vi "MS_Var_to_Comm_Binary.vi"(11 "Boolean":bool) -> (1 "Array":T3[](array[typedef]) {"CROB value"."Control" items=["Nul"=0, "Pulse On"=1, "Pulse Off"=2, "Latch On"=3, "Latch Off"=4, "Close"=65, "Trip"=129]})   [LabVIEW 2016, in "DNP3_Master_Station_Template.lvlib"]
uses:
  DNP3_Master_Station_Template.lvlib
  <vilib>/DNP3/DNP3_Master/Crob With Index.ctl
  <vilib>/DNP3/DNP3_Common/crob.ctl
  <vilib>/DNP3/DNP3_Common/crob_ctrl.ctl
  <vilib>/Utility/file.llb/Read Delimited Spreadsheet (string).vi
  <vilib>/DNP3/DNP3_Common.lvlib
  <vilib>/DNP3/DNP3_Master.lvlib
panel:
  in  "CROB value":T1 {"Control" items=["Nul"=0, "Pulse On"=1, "Pulse Off"=2, "Latch On"=3, "Latch Off"=4, "Close"=65, "Trip"=129]}
  in  "CROB with point index":T3 {"CROB value"."Control" items=["Nul"=0, "Pulse On"=1, "Pulse Off"=2, "Latch On"=3, "Latch Off"=4, "Close"=65, "Trip"=129]}
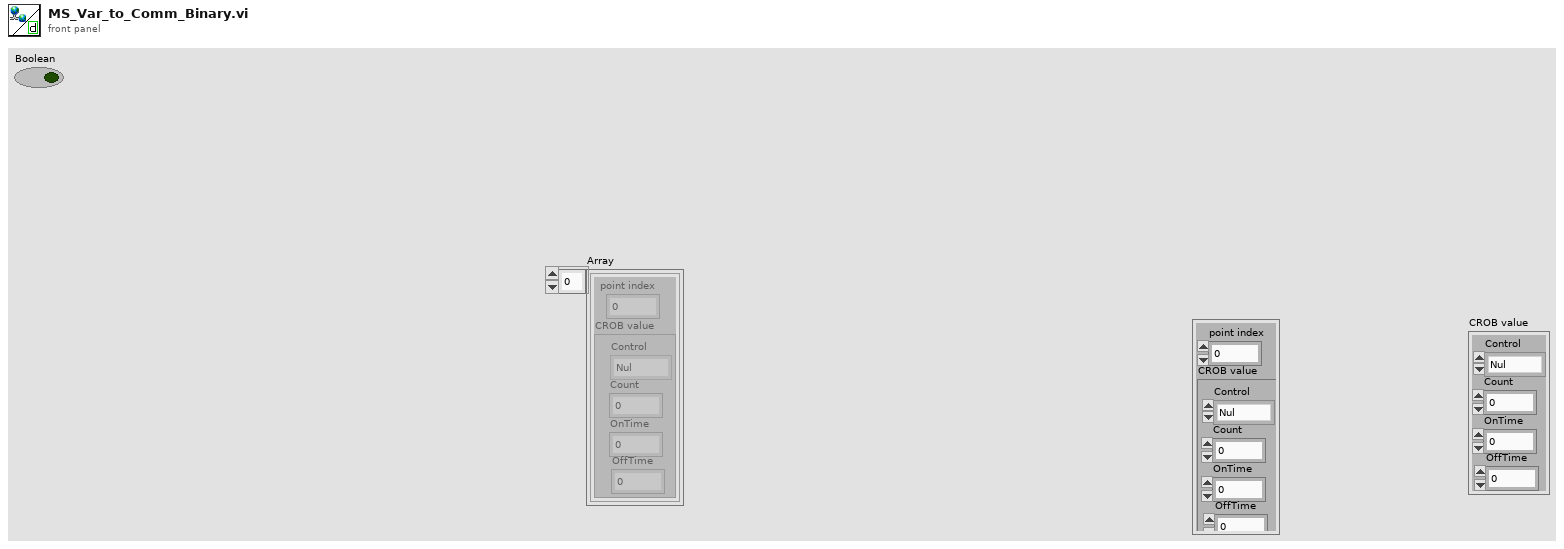
[diagram p1: front panel]
types:
  T1 = typedef "DNP3_Common.lvlib/crob.ctl" = cluster{"OnTime":u32, "Count":u8, "OffTime":u32, "Control":T2}
  T2 = typedef "DNP3_Common.lvlib/crob_ctrl.ctl" = u8
  T3 = typedef "DNP3_Master.lvlib/Crob With Index.ctl" = cluster{"point index":u16, "CROB value":T1}
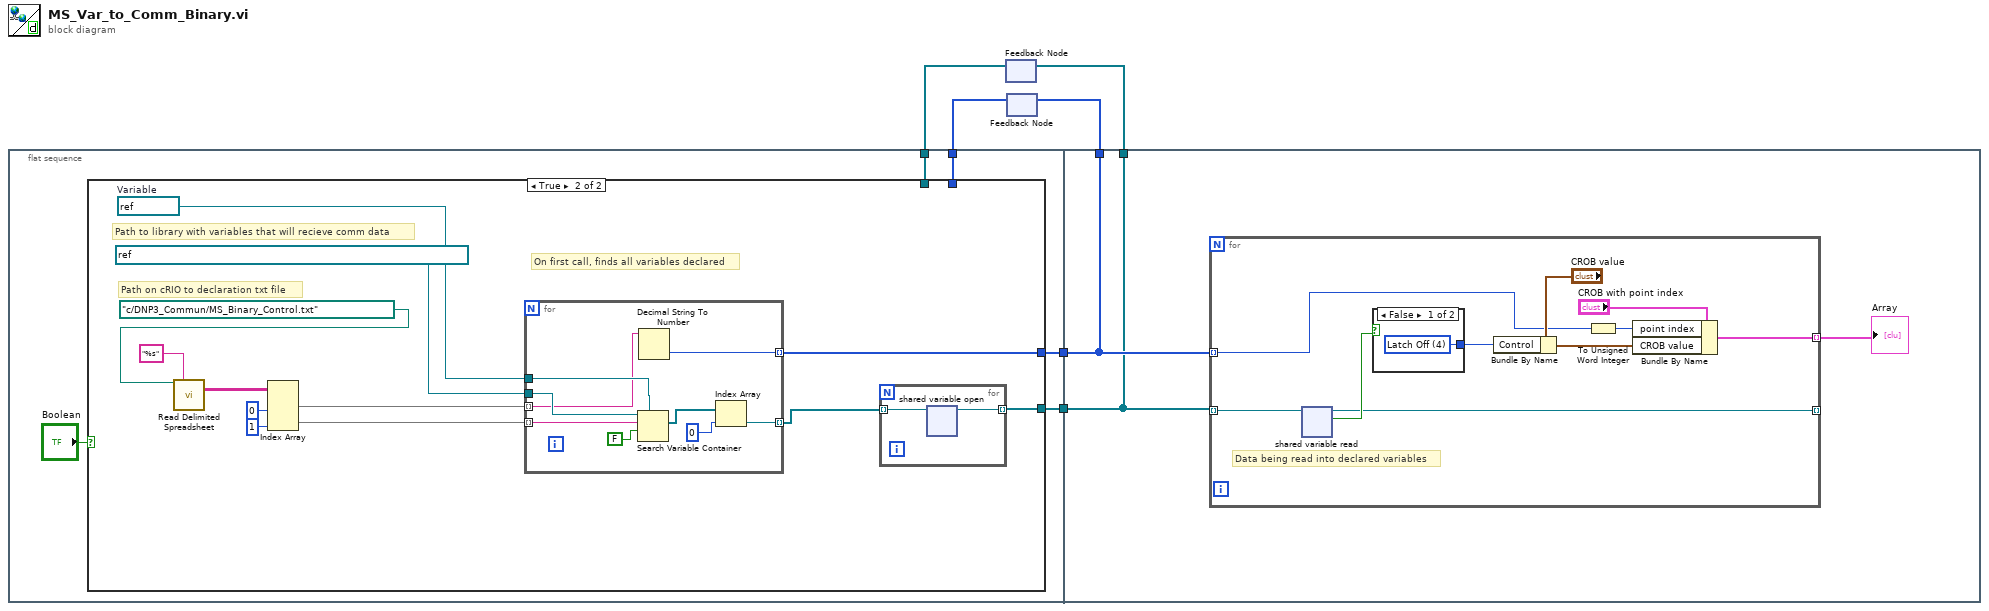
[diagram p0: block diagram]
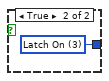
[diagram p3: hidden frame]
diagram:
  n1 = flat-sequence {
    tunnel: [w11] -> w6
    tunnel: [w10] -> w5
    tunnel: w2 -> [w8]
    tunnel: w1 -> [w7]
    tunnel: w6 -> [w37]
    tunnel: w5 -> [w38]
    tunnel: [w38] -> w4
    tunnel: [w37] -> w3
    frame #0 {
      n2 = case shown="True" "Boolean" {
        tunnel: [w12 w14] -> w11
        tunnel: [w13 w16] -> w10
        tunnel: w8 -> [w13 _]
        tunnel: w7 -> [w12 _]
        frame False {
        }
        frame True {
          w17 = refnum<k21> refnum  # Variable
          # "On first call, finds all variables declared"
          # "Path on cRIO to declaration txt file"
          # "Path to library with variables that will recieve comm data"
          n3 = call-poly <vilib>:"Read Delimited Spreadsheet.vi"("file path (dialog if empty)"=path "c:/DNP3_Commun/MS_Binary_Control.txt" ("file path (use dialog)"), "format (%s)"="%s") -> ("all rows"=w21:string[][])  [unwired: 8 in, 5 out]
          n4 = Index Array(array=w21, index (col) #1=0 ("disabled index (col)"), index (col) #2=1 ("index (col)")) -> (element #1=w24:string[], element #2=w25:string[])  [unwired: 2 in]
          n5 = for {
            tunnel: w17 -> [w33]
            tunnel: refnum<k21> "ni.var.psp://localhost/MS_Data_Variables/MS_Binary_Control/" ("container refnum in") -> [w32]
            tunnel: w24 -> [w29] mode=indexing
            tunnel: w25 -> [w31] mode=indexing
            tunnel: [w30] -> w15 mode=indexing
            tunnel: [w28] -> w16 mode=indexing
            n6 = Search Variable Container(7:w33, 9:FALSE, 10:w31, 11:w32) -> (2:w36:refnum<k21>[])  [unwired: 2 in, 2 out]
            n7 = Decimal String To Number(string=w29) -> (number=w28:i32)  [unwired: 2 in, 1 out]
            n8 = Index Array(array=w36, index=0) -> (element=w30:refnum<k21>)
          }
          n9 = for {
            tunnel: w15 -> [w27] mode=indexing
            tunnel: [w26] -> w14 mode=indexing
            n10 = shared-variable-open(w27) -> (w26:refnum<k21>)  [unwired: 2 in, 1 out]
          }
        }
      }
    }
    frame #1 {
      n11 = for {
        tunnel: w37 -> [w44] mode=indexing
        tunnel: [w43] -> _ mode=indexing
        tunnel: [w42] -> w39 mode=indexing
        tunnel: w38 -> [w40] mode=indexing
        # "Data being read into declared variables"
        n12 = shared-variable-read(w44) -> (w43:refnum<k21>, w49:bool)  [unwired: 1 in, 2 out]
        n13 = case shown="False" w49 {
          tunnel: [w50 w51] -> w47
          frame False {
            w50 = T2 4 items=["Nul"=0, "Pulse On"=1, "Pulse Off"=2, "Latch On"=3, "Latch Off"=4, "Close"=65, "Trip"=129] ("Control")
          }
          frame True {
            w51 = T2 3 items=["Nul"=0, "Pulse On"=1, "Pulse Off"=2, "Latch On"=3, "Latch Off"=4, "Close"=65, "Trip"=129] ("Control")
          }
        }
        n14 = Bundle By Name(cluster="CROB value", "Control"=w47) -> (w48:T1)
        n15 = To Unsigned Word Integer(number=w40) -> (unsigned 16bit integer=w41:u16)
        n16 = Bundle By Name(cluster="CROB with point index", "point index"=w41, "CROB value"=w48) -> (w42:T3)
      }
      "Array" <- w39
    }
  }
  n17 = feedback #1() -> (w1:refnum<k21>[])  [unwired: 1 in]
  n18 = feedback-in #1(w3) -> ()
  n19 = feedback-in #2(w4) -> ()
  n20 = feedback #2() -> (w2:i32[])  [unwired: 1 in]
